vi "A-Star Simple Example.vi"() -> ()   [LabVIEW 2015]
uses:
  Defenses.ctl
  <vilib>/Platform/TimedLoop/XDataNode/timing_clust.ctl
  <vilib>/Platform/TimedLoop/XDataNode/nitl_modes.ctl
  <vilib>/Platform/TimedLoop/XDataNode/wakeup.ctl
  <vilib>/Platform/TimedLoop/XDataNode/XDataNode.xnode
  <vilib>/robotics/Navigation/shared/WorldMap/OccupancyGridWorldMap/NI_Robotics_OccupancyGridWorldMap.lvclass
  <vilib>/robotics/Navigation/NI_Robotics_Navigation .lvlib
  <vilib>/Platform/TimedLoop/XDataNode/XDNodeRunTimeDep.lvlib
panel:
  out "Invading":bool
  in  "Inside":bool[][](array[boolean])=[[TRUE, TRUE, TRUE, TRUE, TRUE, TRUE], [TRUE, TRUE, TRUE, TRUE, TRUE, TRUE], [TRUE, TRUE, TRUE, TRUE, TRUE, TRUE], [TRUE, TRUE, TRUE, TRUE, TRUE, TRUE], [TRUE, TRUE, TRUE, TRUE, TRUE, TRUE], [FALSE, FALSE, FALSE, FALSE, FALSE, TRUE], [FALSE, FALSE, FALSE, FALSE, FALSE, FALSE], [FALSE, FALSE, FALSE, FALSE, FALSE, FALSE], [TRUE, FALSE, FALSE, FALSE, FALSE, FALSE], [TRUE, TRUE, TRUE, TRUE, TRUE, TRUE], [TRUE, TRUE, TRUE, TRUE, TRUE, TRUE], [TRUE, TRUE, TRUE, TRUE, TRUE, TRUE], [TRUE, TRUE, TRUE, TRUE, TRUE, TRUE], [TRUE, TRUE, TRUE, TRUE, TRUE, TRUE]]
  in  "Defenses":T2={"Enter"=[100, 100, 50, 20, 100, 100, 80, 10], "Exit"=[100, 100, 50, 20, 5, 10, 80, 10], "Defenses"=[enum."Cheval de Frise", enum."Moat", enum."Ramparts", enum."Drawbridge"], "Positions"=[[1, 9], [2, 9], [3, 9], [4, 9]]}
  in  "Path":cluster{"Start":dbl[], "End":dbl[]}={"Start"=[3.0, 7.0], "End"=[3.0, 11.0]}
  in  "stop":bool
  in  "Ocupancy":bool[][](array[boolean])=[[FALSE, FALSE, TRUE, TRUE, FALSE, TRUE], [FALSE, FALSE, FALSE, FALSE, FALSE, TRUE], [FALSE, FALSE, FALSE, FALSE, FALSE, TRUE], [FALSE, FALSE, FALSE, FALSE, FALSE, TRUE], [TRUE, TRUE, TRUE, TRUE, TRUE, TRUE], [FALSE, FALSE, FALSE, FALSE, FALSE, TRUE], [FALSE, FALSE, FALSE, FALSE, FALSE, FALSE], [FALSE, FALSE, FALSE, FALSE, FALSE, FALSE], [TRUE, FALSE, FALSE, FALSE, FALSE, FALSE], [TRUE, TRUE, TRUE, TRUE, TRUE, TRUE], [TRUE, FALSE, FALSE, FALSE, FALSE, FALSE], [TRUE, FALSE, FALSE, FALSE, FALSE, FALSE], [TRUE, FALSE, FALSE, FALSE, FALSE, FALSE], [TRUE, FALSE, TRUE, TRUE, FALSE, FALSE]]
  out "Intensity Graph":dbl[][](graph)
  # "Portcullis"
  # "Cheval de Frise"
  # "Moat"
  # "Ramparts"
  # "Drawbridge"
  # "Sally port"
  # "Rock wall"
  # "Rough Terrain"
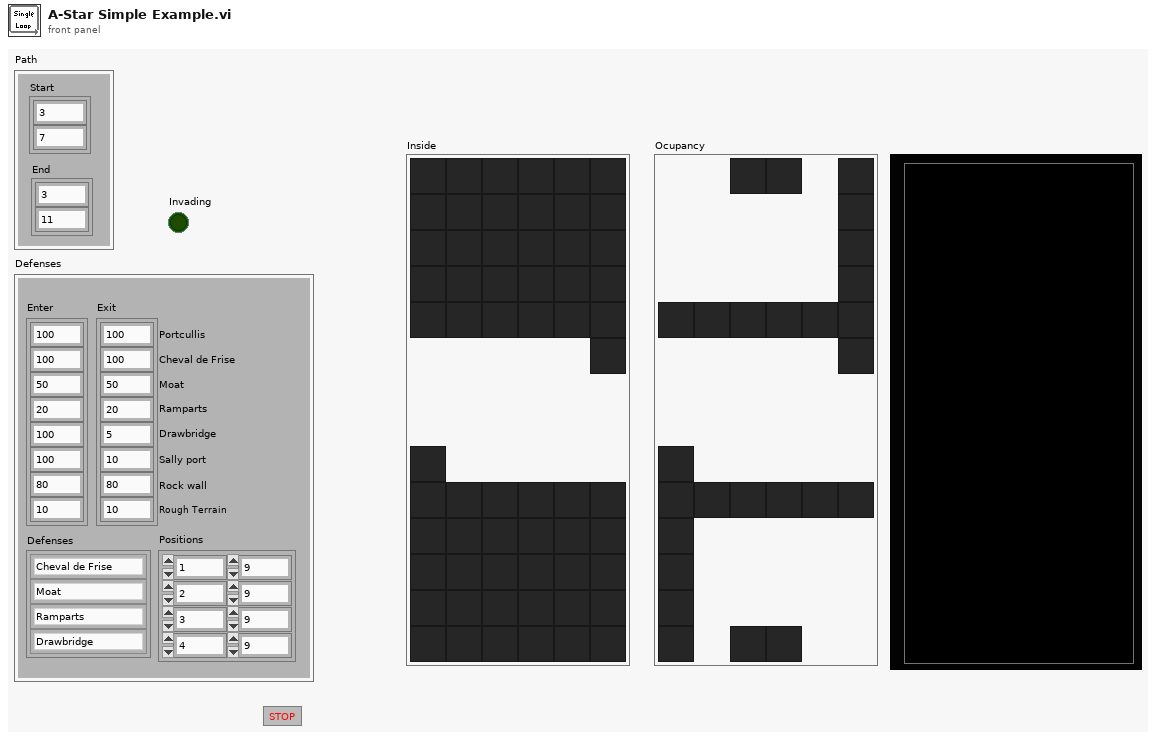
[diagram p1: front panel]
types:
  T1 = typedef "Defenses.ctl" = enum16{"Portcullis", "Cheval de Frise", "Moat", "Ramparts", "Drawbridge", "Sally Port", "Rock Wall", "Rough Terrain", "Low Bar"}
  T2 = cluster{"Enter":i32[], "Exit":i32[], "Defenses":T1[], "Positions":i32[][]}
  T3 = typedef "XDNodeRunTimeDep.lvlib/timing_clust.ctl" = cluster{"Expected End [f-1]":u64, "Actual End [f-1]":u64, "Finished Late? [f-1]":bool, "Expected End [i-1]":u64, "Actual End [i-1]":u64, "Finished Late? [i-1]":bool, "Expected Start [i]":u64, "Actual Start [i]":u64, "Expected Start [f]":u64, "Actual Start [f]":u64, "Source Name":string, "Structure Name":string, "Period":i64, "Deadline":i64, "Offset":i64, "Start":i64, "Priority":i32, "Timeout":i32, "Mode":T4, "Wakeup Reason":T5, "Error":errorcluster, "Source Type":string, "Secondary Source Type":string, "Global End Time":u64, "Global Start Time":u64, "Frame Duration":u64, "Iteration Duration":u64, "Assigned CPU":i32, "I/O Scan Engine Mode":u32}
  T4 = typedef "XDNodeRunTimeDep.lvlib/nitl_modes.ctl" = enum32{"No Change", "Process missed periods, maintain original phase", "Discard missed periods, maintain original phase", "Process missed periods, ignore original phase", "Discard missed periods, ignore original phase"}
  T5 = typedef "XDNodeRunTimeDep.lvlib/wakeup.ctl" = enum32{"Normal", "Aborted", "Asynchronous wakeup", "Timing source error", "Timed loop error", "Timeout"}
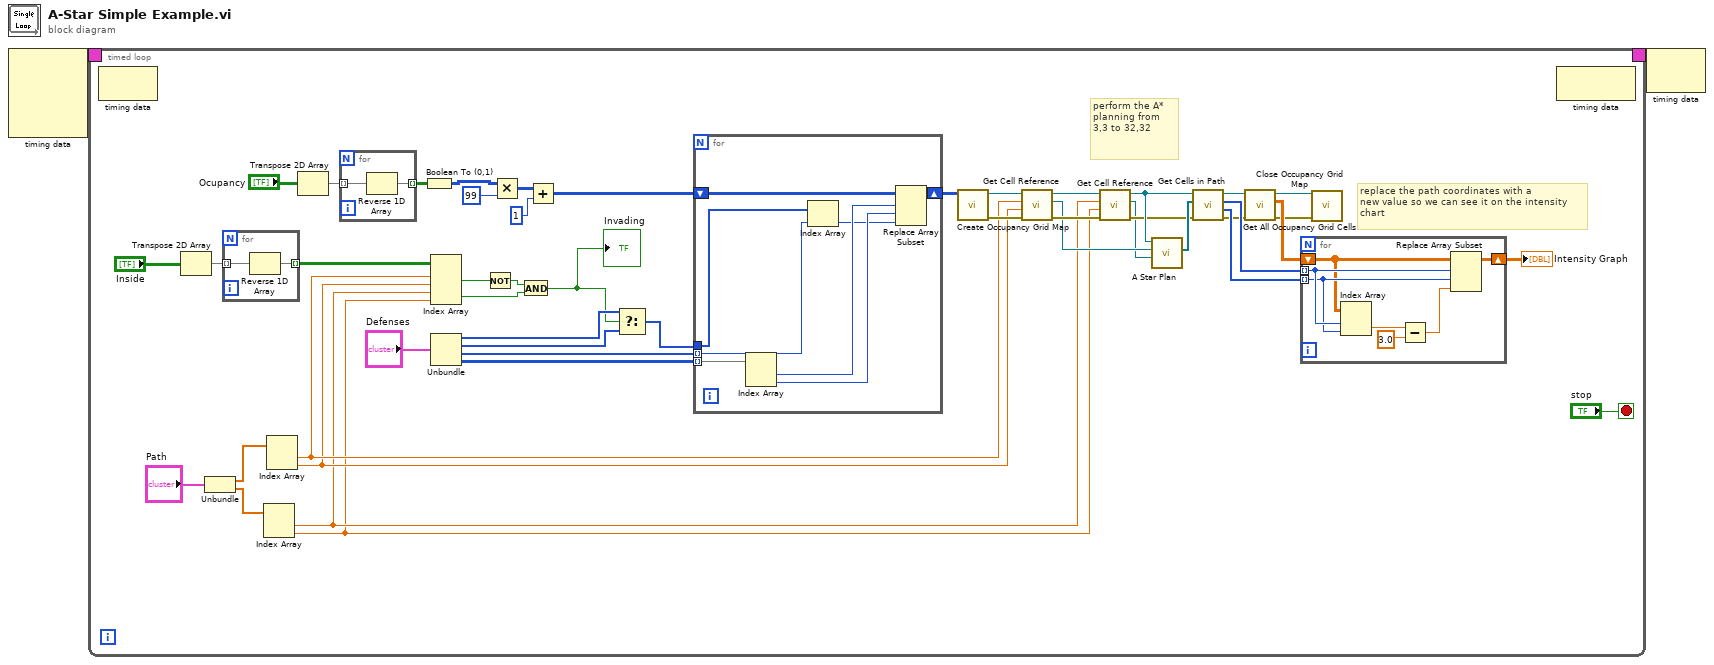
[diagram p0: block diagram]
diagram:
  n1 = node-c288() -> (w2:T3)  [unwired: 4 in]
  n2 = timed-loop {
    timing: w2 -> [_]
    timing-out: [_] -> w1
    stop <- "stop" stop-if-true
    # "replace the path coordinates with a\nnew value so we can see it on the intensity \nchart"
    # "perform the A* planning from 3,3 to 32,32"
    n3 = node-c288() -> ()  [unwired: 1 in, 1 out]
    n4 = Transpose 2D Array(2D array="Inside") -> (transposed array=w10:bool[][])
    n5 = Unbundle("Path") -> ("Start"=w23:dbl[], "End"=w22:dbl[])
    n6 = for {
      tunnel: w10 -> [w51] mode=indexing
      tunnel: [w50] -> w8 mode=indexing
      n7 = Reverse 1D Array(array=w51) -> (reversed array=w50:bool[])
    }
    n8 = Index Array(array=w22) -> (element #1=w5:dbl, element #2=w4:dbl)  [unwired: 2 in]
    n9 = Index Array(array=w23) -> (element #1=w7:dbl, element #2=w6:dbl)  [unwired: 2 in]
    n10 = Transpose 2D Array(2D array="Ocupancy") -> (transposed array=w40:bool[][])
    n11 = for {
      tunnel: w40 -> [w63] mode=indexing
      tunnel: [w62] -> w39 mode=indexing
      n12 = Reverse 1D Array(array=w63) -> (reversed array=w62:bool[])
    }
    n13 = Boolean To (0,1)(Boolean=w39) -> (0, 1=w25:i16[][])
    n14 = Index Array(array=w8, index (row) #1=w7, index (col) #1=w6, index (row) #2=w5, index (col) #2=w4) -> (element #1=w13:bool, element #2=w11:bool)
    n15 = Unbundle("Defenses") -> ("Enter"=w14:i32[], "Exit"=w15:i32[], "Defenses"=w17:T1[], "Positions"=w18:i32[][])
    n16 = Not(x=w13) -> (.not. x?=w12:bool)
    n17 = Multiply(x=w25, y=99) -> (x*y=w38:i32[][])
    n18 = And(x=w12, y=w11) -> (x .and. y?=w3:bool)
    "Invading" <- w3
    n19 = Add(x=w38, y=1) -> (x+y=w21:i32[][])
    n20 = Select(t=w14, s=w3, f=w15) -> (s? t:f=w16:i32[])
    n21 = for {
      tunnel: w17 -> [w55] mode=indexing
      tunnel: w16 -> [w56]
      tunnel: w18 -> [w59] mode=indexing
      shift-right: [w57] -> w19
      shift-left: w21 -> [w58]
      n22 = Index Array(array=w59) -> (element #1=w54:i32, element #2=w53:i32)  [unwired: 2 in]
      n23 = Index Array(array=w56, index=w55) -> (element=w52:i32)
      n24 = Replace Array Subset(array=w58, new element=w52, index (row)=w54, index (col)=w53) -> (w57:i32[][])
    }
    n25 = call <vilib>:"Create Occupancy Grid Map.vi"("occupancy grid"=w19) -> ("error out"=w36:errorcluster, "map reference out"=w29:refnum<data-value>)  [unwired: 9 in]
    n26 = call <vilib>:"Get Cell Reference.vi"("error in (no error)"=w36, "y"=w6, "x"=w7, "map reference in"=w29) -> ("error out"=w35:errorcluster, "cell reference"=w30:refnum<data-value>, "map reference out"=w49:refnum<data-value>)  [unwired: 4 in, 1 out]
    n27 = call <vilib>:"Get Cell Reference.vi"("error in (no error)"=w35, "y"=w4, "x"=w5, "map reference in"=w49) -> ("error out"=w34:errorcluster, "cell reference"=w28:refnum<data-value>, "map reference out"=w47:refnum<data-value>)  [unwired: 4 in, 1 out]
    n28 = call <vilib>:"A Star Plan.vi"("goal reference"=w28, "start reference"=w30, "map reference in"=w47) -> ("path references"=w48:refnum<data-value>[])  [unwired: 5 in, 3 out]
    n29 = call <vilib>:"Get Cells in Path.vi"("error in (no error)"=w34, "path references"=w48, "map reference in"=w47) -> ("error out"=w33:errorcluster, "y coordinates"=w44:i32[], "x coordinates"=w43:i32[], "map reference out"=w46:refnum<data-value>)  [unwired: 5 in]
    n30 = call <vilib>:"Get All Occupancy Grid Cells.vi"("error in (no error)"=w33, "map reference in"=w46) -> ("error out"=w32:errorcluster, "occupancy grid"=w45:dbl[][], "map reference out"=w27:refnum<data-value>)  [unwired: 7 in]
    n31 = for {
      tunnel: w44 -> [w68] mode=indexing
      tunnel: w43 -> [w69] mode=indexing
      shift-right: [w70] -> w42
      shift-left: w45 -> [w64]
      n32 = Index Array(array=w64, index (row)=w69, index (col)=w68) -> (element=w67:dbl)
      n33 = Subtract(x=w67, y=3.0) -> (x-y=w66:dbl)
      n34 = Replace Array Subset(array=w64, new element=w66, index (row)=w69, index (col)=w68) -> (w70:dbl[][])
    }
    "Intensity Graph" <- w42
    n35 = call <vilib>:"Close Occupancy Grid Map.vi"("error in (no error)"=w32, "map reference in"=w27) -> ()  [unwired: 9 in, 1 out]
    n36 = node-c288() -> ()  [unwired: 1 in, 1 out]
  }
  n37 = node-c288(w1) -> ()  [unwired: 1 out]
